vi "Get value string.vi"(8 "error in (no error)":errorcluster, 11 "Column in":refnum<class "Column Parent.lvclass">) -> (0 "error out":errorcluster, 2 "Value":string, 3 "Column out":refnum<class "Column Parent.lvclass">)   [LabVIEW 2020, in "Basic Columns.lvlib" / "Column Parent.lvclass"]
uses:
  Column Parent.lvclass
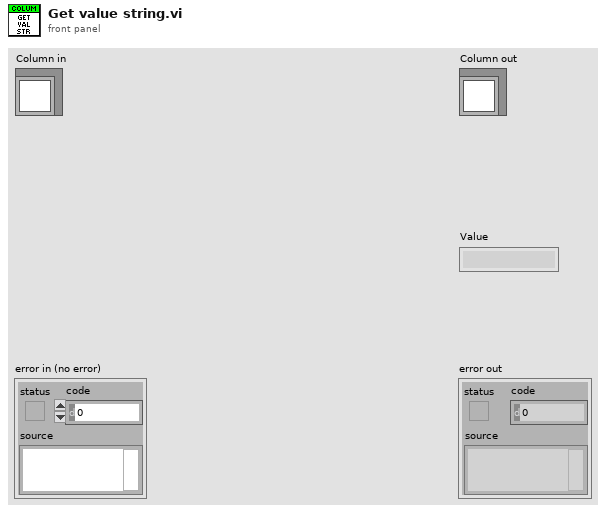
[diagram p1: front panel]
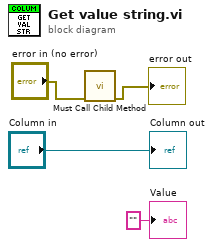
[diagram p0: block diagram]
diagram:
  n1 = call "Must Call Child Method.vi"("error in"="error in (no error)") -> ("error out"=→"error out":errorcluster)  [unwired: 10 in]
  "Column out" <- "Column in"
  "Value" <- "" ("Value")
